vi "RefreshRequestSummaryinRoom.vi"(8 "error in (no error)":errorcluster, 10 "Room":string) -> (0 "error out":errorcluster, 2 "Fresh Room":string)   [LabVIEW 2015]
uses:
  TypeDef/RequestActionEnum.ctl
  LVClasses/Room/Room.lvclass/Room.ctl
  LVClasses/Request/Request.lvclass/Request.ctl
  LVClasses/Request/Read Summary.vi
  LVClasses/Room/Read Room Number.vi
  LVClasses/Room/Write RoomRequests.vi
  LVClasses/Room/Room.lvclass
  LVClasses/Request/Request.lvclass
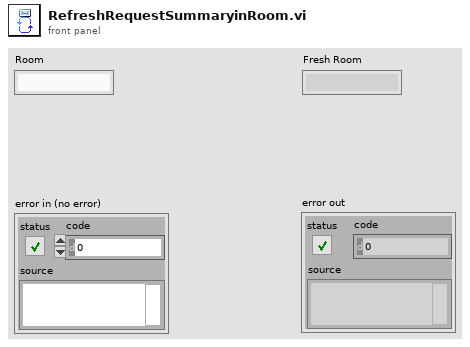
[diagram p1: front panel]
types:
  T1 = typedef "RequestActionEnum.ctl" = enum16{"Init", "ReadRequests", "ReadRequest", "AddRequest", "RemoveRequest", "ToDisk", "Ack", "Complete", "CheckAlarms", "PIntoRoom", "Read Summary", "GetRequestForRoom"}
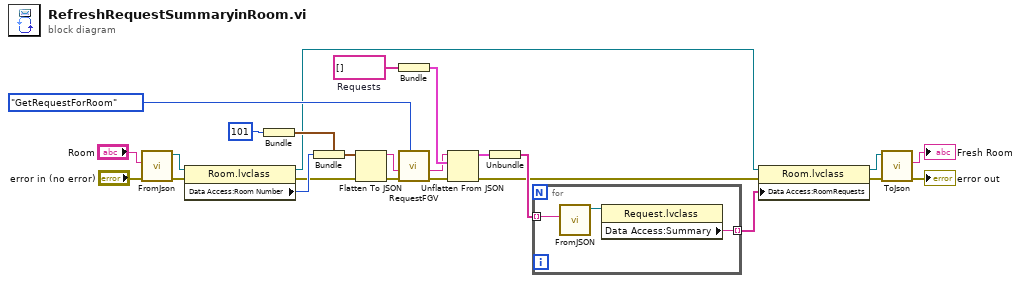
[diagram p0: block diagram]
diagram:
  w17 = string[] []  # Requests
  n1 = call "FromJson.vi"("error in (no error)"="error in (no error)", "String"="Room") -> ("error out"=w5:errorcluster, "Room out"=w23:refnum<class "Room.lvclass">)  [unwired: 8 in]
  n2 = property class="Room.lvclass"(reference=w23, error in=w5) -> (reference out=w12:refnum<class "Room.lvclass">, error out=w4:errorcluster, "Data Access:Room Number"=w19:i32)
  n3 = Bundle("Room"=101) -> (w21:cluster{"Room":i32})  [unwired: 1 in]
  n4 = Bundle(cluster=w21, "Room"=w19) -> (w20:cluster{"Room":i32})
  n5 = Flatten To JSON(anything=w20, error in (no error)=w4) -> (JSON string=w18:string, 11:w3:errorcluster)  [unwired: 1 in]
  n6 = Bundle("Requests"=w17) -> (w16:cluster{"Requests":string[]})  [unwired: 1 in]
  n7 = call "RequestFGV.vi"("Actions"=RequestActionEnum."GetRequestForRoom", "error in (no error)"=w3, "Data In"=w18) -> ("error out"=w2:errorcluster, "Data Out"=w14:string)  [unwired: 7 in]
  n8 = Unflatten From JSON(JSON string=w14, type and defaults=w16, error in (no error)=w2) -> (value=w15:cluster{"Requests":string[]}, error out=w1:errorcluster)  [unwired: 4 in]
  n9 = Unbundle(w15) -> ("Requests"=w13:string[])
  n10 = for {
    tunnel: w13 -> [w28] mode=indexing
    tunnel: [w26] -> w10 mode=indexing
    n11 = call "FromJSON.vi"("Request"=w28) -> ("Request out"=w27:refnum<class "Request.lvclass">)  [unwired: 9 in, 1 out]
    n12 = property class="Request.lvclass"(reference=w27) -> ("Data Access:Summary"=w26:string)  [unwired: 1 in, 2 out]
  }
  n13 = property class="Room.lvclass"(reference=w12, error in=w1, "Data Access:RoomRequests"=w10) -> (reference out=w11:refnum<class "Room.lvclass">, error out=w9:errorcluster)
  n14 = call "ToJson.vi"("error in (no error)"=w9, "Room in"=w11) -> ("error out"=→"error out":errorcluster, "String"=→"Fresh Room":string)  [unwired: 7 in, 1 out]
